vi "Exponential Growth And Dead Zone.vi"(1 "Dead Zone":dbl, 2 "Joy Stick Input":dbl, 3 "Power":dbl) -> (0 "Fixed Output":dbl)   [LabVIEW 2013]
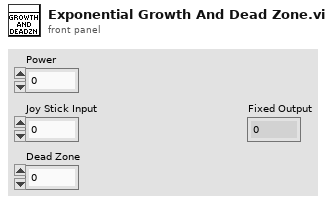
[diagram p1: front panel]
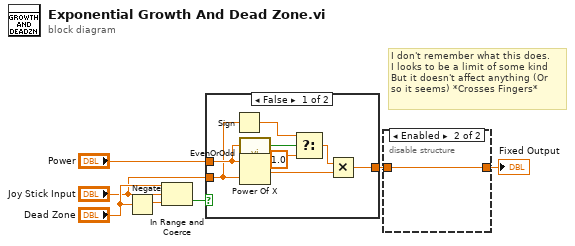
[diagram p0: block diagram]
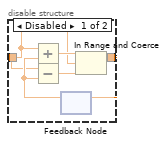
[diagram p2: hidden frame]
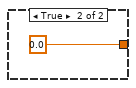
[diagram p3: hidden frame]
diagram:
  # "I don't remember what this does.\nI looks to be a limit of some kind\nBut it doesn't affect anything (Or\nso it seems) *Crosses Fingers*"
  n1 = Negate(x="Dead Zone") -> (-x=w7:dbl)
  n2 = In Range and Coerce(upper limit="Dead Zone", x="Joy Stick Input", lower limit=w7) -> (In Range?=w5:bool)  [unwired: 1 out]
  n3 = case shown="False" w5 {
    tunnel: "Joy Stick Input" -> [w12 _]
    tunnel: "Power" -> [w15 _]
    tunnel: [w8 0.0] -> w1
    frame False {
      n4 = Sign(1:w12) -> (0:w13:dbl)
      n5 = call "EvenOrOdd.vi"("Number"=w15) -> ("Even(T) or Odd(F)"=w14:bool)  [unwired: 2 in]
      n6 = Power Of X(1:w12, 2:w15) -> (0:w9:dbl)
      n7 = Select(t=w13, s=w14, f=1.0) -> (s? t:f=w10:dbl)
      n8 = Multiply(x=w10, y=w9) -> (x*y=w8:dbl)
    }
    frame True {
    }
  }
  n9 = disable-structure shown="Enabled" {
    disable-tunnel: [w19 w22] -> w2
    disable-tunnel: w1 -> [w17 w22]
    frame Disabled {
      n10 = feedback #1() -> (w18:dbl)  [unwired: 1 in]
      n11 = Add(x=w17, y=w18) -> (x+y=w20:dbl)
      n12 = Subtract(x=w17, y=w18) -> (x-y=w21:dbl)
      n13 = In Range and Coerce(upper limit=w20, x=w17, lower limit=w21) -> (coerced(x)=w19:dbl)  [unwired: 1 out]
      n14 = feedback-in #1(w19) -> ()
    }
    frame Enabled {
    }
  }
  "Fixed Output" <- w2
